vi "Dual XDCR AttnScan.vi"(0 "Length of\none plane (mm)":refnum<vi>, 1 "Distance between\nscan lines (um)":refnum<vi>, 3 "Case Name":refnum<vi>, 4 "DBSP2":refnum<vi>, 5 "DBSP1":refnum<vi>, 8 "Length of\nall planes (mm)":refnum<vi>, 9 "Scan Size":refnum<vi>, 10 "Length of Z Scan (mm)":dbl=5.0 format="%#_13g", 11 "Distance between\nZ planes (um)":i32=100, 12 "scan pair":T1=enum."y-(z) scan", 13 "Transducer":refnum<vi>, 14 "Attenuation Scan":bool, 15 "DBSP1":sgl, 17 "DBSP2":sgl, 19 "Dual XDCR Settings in":T2 {"XDCR Settings"."UT340 Controls"."Low Pass Filter (MHz)" min=-6 max=60 step=1; "XDCR Settings"."UT340 Controls"."High Pass Filter (MHz)" min=1 max=20 step=1; "XDCR Settings"."UT340 Controls"."Rep Rate (Hz)" min=20 step=1; "XDCR Settings"."UT340 Controls"."Pulse Width (ns)" min=100.0 max=250.0 step=2.0; "XDCR Settings"."UT340 Controls"."Voltage" min=100 max=250 step=2; "XDCR Settings"."UT340 Controls"."PC Gain (dB)" min=2 max=72; "XDCR Settings"."UT340 Controls"."PE Gain (dB)" min=-6 max=60 step=1; "XDCR Settings"."JSR Complete"."JSR Trigger Settings"."PRF (Hz)" items=["100 Hz"=0.1, "200 Hz"=0.2, "400 Hz"=0.4, "600 Hz"=0.6, "800 Hz"=0.8, "1000 Hz"=1.0, "1250 Hz"=1.25, "1500 Hz"=1.5, "1750 Hz"=1.75, "2000 Hz"=2.0, "2500 Hz"=2.5, "3000 Hz"=3.0, "3500 Hz"=3.5, "4000 Hz"=4.0, "4500 Hz"=4.5, "5000 Hz"=5.0]; "XDCR Settings"."JSR Complete"."JSR Trigger Settings"."Trigger Source" items=["Internal", "External"]; "XDCR Settings"."JSR Complete"."JSR Trigger Settings"."External Trigger Limit" items=["No Limit", "5 kHz"]; "XDCR Settings"."JSR Complete"."JSR Receive Settings"."Gain (dB)" min=-13 max=66 step=1; "XDCR Settings"."JSR Complete"."JSR Receive Settings"."Low Pass Filter" items=["5 MHz"=5, "10 MHz"=10, "15 MHz"=15, "22.5 MHz"=22, "35 MHz"=35, "50 MHz"=50]; "XDCR Settings"."JSR Complete"."JSR Receive Settings"."High Pass Filter" items=["DC"=0, "1 MHz"=1000, "2.5 MHz"=2500, "5 MHz"=5000, "7.5 MHz"=7500, "12.5 MHz"=12500]; "XDCR Settings"."JSR Complete"."JSR Receive Settings"."Receiver Mode" items=["Echo", "Through"]; "XDCR Settings"."JSR Complete"."JSR Pulse Settings"."Pulser Voltage (V)" items=["100"=100, "125"=125, "150"=150, "175"=175, "200"=200, "225"=225, "250"=250, "275"=275, "300"=300, "325"=325, "350"=350, "375"=375, "400"=400, "425"=425, "450"=450, "475"=475]; "XDCR Settings"."JSR Complete"."JSR Pulse Settings"."Pulser Impedance" items=["High z", "Low z"]; "XDCR Settings"."JSR Complete"."JSR Pulse Settings"."Pulse Energy Level" items=["0 (Minimum)", "1", "2", "3 (Maximum)"]; "XDCR Settings"."JSR Complete"."JSR Pulse Settings"."Damping" items=["331 Ohms"=331, "198 Ohms"=198, "142 Ohms"=142, "110 Ohms"=110, "92 Ohms"=92, "77 Ohms"=77, "67 Ohms"=67, "59 Ohms"=59, "52 Ohms"=52, "47 Ohms"=47, "43 Ohms"=43, "39 Ohms"=39, "37 Ohms"=37, "34 Ohms"=34, "32 Ohms"=32, "30 Ohms"=30]; "XDCR Settings"."Panametrics Settings"."FINE ATTENUATION" items=["00.0", "00.5", "01.0", "01.5", "02.0", "02.5", "03.0", "03.5", "04.0", "04.5", "05.0", "05.5", "06.0", "06.5", "07.0", "07.5", "08.0", "08.5", "09.0", "09.5", "10.0", "10.5", "11.0", "11.5", "12.0", "12.5", "13.0", "13.5", "14.0", "14.5", "15.0", "15.5"]; "XDCR Settings"."Panametrics Settings"."COARSE ATTENUATION" items=["00.0", "10.0", "20.0", "30.0", "40.0", "50.0"]; "XDCR Settings"."Panametrics Settings"."GAIN (db)" items=["26.0", "40.0", "54.0"]; "XDCR Settings"."Panametrics Settings"."PRF (KHz)" items=["XREMT", "EXBNC", "0.200", "0.500", "1.000", "2.000", "5.000", "10.00", "20.00"]; "XDCR Settings"."Panametrics Settings"."MODE" items=["P/ E", "THRU", "RPP", "EXT_PLSR"]; "XDCR Settings"."Panametrics Settings"."LP FILT (MHz)" items=["20", "50", "100", "200"]; "XDCR Settings"."Panametrics Settings"."HP FILT (KHz)" items=["1", "1000", "3000", "10000"]; "XDCR Settings"."Panametrics Settings"."DAMPING (Ohm)" items=["7", "10", "16", "20", "26", "30", "40", "50"]; "XDCR Settings"."Panametrics Settings"."ENERGY (uJ)" items=["1", "2", "4", "8", "16", "32"]; "XDCR Settings"."Daxsonics Settings"."Freq (MHz)" items=["4"=4, "5"=5, "6"=6, "8"=8, "10"=10, "12"=12, "14"=14, "15"=15, "16"=16, "17"=17, "18"=18, "20"=20, "25"=25, "30"=30, "35"=35, "40"=40, "45"=45, "50"=50]; "XDCR Settings"."Daxsonics Settings"."Voltage (V)" items=["0"=0, "5"=5, "10"=10, "15"=15, "20"=20, "25"=25, "30"=30, "35"=35, "40"=40, "45"=45, "50"=50, "55"=55, "60"=60, "65"=65, "70"=70, "75"=75, "80"=80, "85"=85, "90"=90, "95"=95, "100"=100, "110"=110, "120"=120, "130"=130, "140"=140, "150"=150, "160"=160, "170"=170, "180"=180, "190"=190]; "XDCR Settings"."Daxsonics Settings"."Gain (dB)" items=["22"=22, "25"=25, "28"=28, "31"=31, "34"=34, "37"=37, "40"=40, "43"=43, "46"=46, "49"=49, "52"=52, "55"=55, "58"=58, "61"=61, "64"=64, "67"=67]; "XDCR Settings"."Digitizer Settings"."Additional dig delay (ms)" format="%.2f"; "XDCR Settings"."Digitizer Settings"."Time scale per Div" items=["100 ns"=0.1, "200 ns"=0.2, "500 ns"=0.5, "1 micros"=1.0, "2 micros"=2.0, "5 micros"=5.0, "10 micros"=10.0, "20 micros"=20.0, "50 micros"=50.0, "100 micros"=100.0, "200 micros"=200.0, "500 micros"=500.0, "1 ms"=1000.0, "2 ms"=2000.0, "5 ms"=5000.0, "10 ms"=10000.0, "20 ms"=20000.0, "50 ms"=50000.0, "100 ms"=100000.0, "200 ms"=200000.0]; "XDCR Settings"."Digitizer Settings"."RF data Sampling"."rf points per line" min=1; "XDCR Settings"."Digitizer Settings"."RF data Sampling"."Ref Delay (ms)" format="%.2f"}) -> (16 "scan pair out":T1, 20 "lines per plane":dbl, 21 "Distance between\nscan lines (um)":sgl, 23 "number of planes":dbl, 24 "Distance between\nscan planes (um)":sgl, 25 "Dual XDCR Settings out":T2 {"XDCR Settings"."UT340 Controls"."Low Pass Filter (MHz)" min=-6 max=60 step=1; "XDCR Settings"."UT340 Controls"."High Pass Filter (MHz)" min=1 max=20 step=1; "XDCR Settings"."UT340 Controls"."Rep Rate (Hz)" min=20 step=1; "XDCR Settings"."UT340 Controls"."Pulse Width (ns)" min=100.0 max=250.0 step=2.0; "XDCR Settings"."UT340 Controls"."Voltage" min=100 max=250 step=2; "XDCR Settings"."UT340 Controls"."PC Gain (dB)" min=2 max=72; "XDCR Settings"."UT340 Controls"."PE Gain (dB)" min=-6 max=60 step=1; "XDCR Settings"."JSR Complete"."JSR Trigger Settings"."PRF (Hz)" items=["100 Hz"=0.1, "200 Hz"=0.2, "400 Hz"=0.4, "600 Hz"=0.6, "800 Hz"=0.8, "1000 Hz"=1.0, "1250 Hz"=1.25, "1500 Hz"=1.5, "1750 Hz"=1.75, "2000 Hz"=2.0, "2500 Hz"=2.5, "3000 Hz"=3.0, "3500 Hz"=3.5, "4000 Hz"=4.0, "4500 Hz"=4.5, "5000 Hz"=5.0]; "XDCR Settings"."JSR Complete"."JSR Trigger Settings"."Trigger Source" items=["Internal", "External"]; "XDCR Settings"."JSR Complete"."JSR Trigger Settings"."External Trigger Limit" items=["No Limit", "5 kHz"]; "XDCR Settings"."JSR Complete"."JSR Receive Settings"."Gain (dB)" min=-13 max=66 step=1; "XDCR Settings"."JSR Complete"."JSR Receive Settings"."Low Pass Filter" items=["5 MHz"=5, "10 MHz"=10, "15 MHz"=15, "22.5 MHz"=22, "35 MHz"=35, "50 MHz"=50]; "XDCR Settings"."JSR Complete"."JSR Receive Settings"."High Pass Filter" items=["DC"=0, "1 MHz"=1000, "2.5 MHz"=2500, "5 MHz"=5000, "7.5 MHz"=7500, "12.5 MHz"=12500]; "XDCR Settings"."JSR Complete"."JSR Receive Settings"."Receiver Mode" items=["Echo", "Through"]; "XDCR Settings"."JSR Complete"."JSR Pulse Settings"."Pulser Voltage (V)" items=["100"=100, "125"=125, "150"=150, "175"=175, "200"=200, "225"=225, "250"=250, "275"=275, "300"=300, "325"=325, "350"=350, "375"=375, "400"=400, "425"=425, "450"=450, "475"=475]; "XDCR Settings"."JSR Complete"."JSR Pulse Settings"."Pulser Impedance" items=["High z", "Low z"]; "XDCR Settings"."JSR Complete"."JSR Pulse Settings"."Pulse Energy Level" items=["0 (Minimum)", "1", "2", "3 (Maximum)"]; "XDCR Settings"."JSR Complete"."JSR Pulse Settings"."Damping" items=["331 Ohms"=331, "198 Ohms"=198, "142 Ohms"=142, "110 Ohms"=110, "92 Ohms"=92, "77 Ohms"=77, "67 Ohms"=67, "59 Ohms"=59, "52 Ohms"=52, "47 Ohms"=47, "43 Ohms"=43, "39 Ohms"=39, "37 Ohms"=37, "34 Ohms"=34, "32 Ohms"=32, "30 Ohms"=30]; "XDCR Settings"."Panametrics Settings"."FINE ATTENUATION" items=["00.0", "00.5", "01.0", "01.5", "02.0", "02.5", "03.0", "03.5", "04.0", "04.5", "05.0", "05.5", "06.0", "06.5", "07.0", "07.5", "08.0", "08.5", "09.0", "09.5", "10.0", "10.5", "11.0", "11.5", "12.0", "12.5", "13.0", "13.5", "14.0", "14.5", "15.0", "15.5"]; "XDCR Settings"."Panametrics Settings"."COARSE ATTENUATION" items=["00.0", "10.0", "20.0", "30.0", "40.0", "50.0"]; "XDCR Settings"."Panametrics Settings"."GAIN (db)" items=["26.0", "40.0", "54.0"]; "XDCR Settings"."Panametrics Settings"."PRF (KHz)" items=["XREMT", "EXBNC", "0.200", "0.500", "1.000", "2.000", "5.000", "10.00", "20.00"]; "XDCR Settings"."Panametrics Settings"."MODE" items=["P/ E", "THRU", "RPP", "EXT_PLSR"]; "XDCR Settings"."Panametrics Settings"."LP FILT (MHz)" items=["20", "50", "100", "200"]; "XDCR Settings"."Panametrics Settings"."HP FILT (KHz)" items=["1", "1000", "3000", "10000"]; "XDCR Settings"."Panametrics Settings"."DAMPING (Ohm)" items=["7", "10", "16", "20", "26", "30", "40", "50"]; "XDCR Settings"."Panametrics Settings"."ENERGY (uJ)" items=["1", "2", "4", "8", "16", "32"]; "XDCR Settings"."Daxsonics Settings"."Freq (MHz)" items=["4"=4, "5"=5, "6"=6, "8"=8, "10"=10, "12"=12, "14"=14, "15"=15, "16"=16, "17"=17, "18"=18, "20"=20, "25"=25, "30"=30, "35"=35, "40"=40, "45"=45, "50"=50]; "XDCR Settings"."Daxsonics Settings"."Voltage (V)" items=["0"=0, "5"=5, "10"=10, "15"=15, "20"=20, "25"=25, "30"=30, "35"=35, "40"=40, "45"=45, "50"=50, "55"=55, "60"=60, "65"=65, "70"=70, "75"=75, "80"=80, "85"=85, "90"=90, "95"=95, "100"=100, "110"=110, "120"=120, "130"=130, "140"=140, "150"=150, "160"=160, "170"=170, "180"=180, "190"=190]; "XDCR Settings"."Daxsonics Settings"."Gain (dB)" items=["22"=22, "25"=25, "28"=28, "31"=31, "34"=34, "37"=37, "40"=40, "43"=43, "46"=46, "49"=49, "52"=52, "55"=55, "58"=58, "61"=61, "64"=64, "67"=67]; "XDCR Settings"."Digitizer Settings"."Additional dig delay (ms)" format="%.2f"; "XDCR Settings"."Digitizer Settings"."Time scale per Div" items=["100 ns"=0.1, "200 ns"=0.2, "500 ns"=0.5, "1 micros"=1.0, "2 micros"=2.0, "5 micros"=5.0, "10 micros"=10.0, "20 micros"=20.0, "50 micros"=50.0, "100 micros"=100.0, "200 micros"=200.0, "500 micros"=500.0, "1 ms"=1000.0, "2 ms"=2000.0, "5 ms"=5000.0, "10 ms"=10000.0, "20 ms"=20000.0, "50 ms"=50000.0, "100 ms"=100000.0, "200 ms"=200000.0]; "XDCR Settings"."Digitizer Settings"."RF data Sampling"."rf points per line" min=1; "XDCR Settings"."Digitizer Settings"."RF data Sampling"."Ref Delay (ms)" format="%.2f"})   [LabVIEW 2022 SP3]
uses:
  Dual XDCR Complete Settings.ctl
  XDCRSettings.ctl
  Pulsers/Daxsonics/-DaxSubroutines/Dax_Control_Cluster.ctl
  Pulsers/Panametrics/Pana5900.ctl
  Pulsers/JSR/Controls/JSR Complete.ctl
  Pulsers/JSR/Controls/JSR Pulse.ctl
  Pulsers/JSR/Controls/Damping.ctl
  Pulsers/JSR/Controls/Energy.ctl
  Pulsers/JSR/Controls/Z.ctl
  Pulsers/JSR/Controls/Volt.ctl
  Pulsers/JSR/Controls/JSR Recieve.ctl
  Pulsers/JSR/Controls/Mode.ctl
  Pulsers/JSR/Controls/HPF.ctl
  Pulsers/JSR/Controls/LPF.ctl
  Pulsers/JSR/Controls/Gain.ctl
  Pulsers/JSR/Controls/JSR Trigger.ctl
  Pulsers/JSR/Controls/Trig Limit.ctl
  Pulsers/JSR/Controls/Trig Source.ctl
  Pulsers/JSR/Controls/PRF.ctl
  Pulsers/UTEX/Controls/UTEX Controls.ctl
  Motion Controllers/-MotionRoutines/ScanAxis.ctl
  <vilib>/regexp/Match Regular Expression.xnode
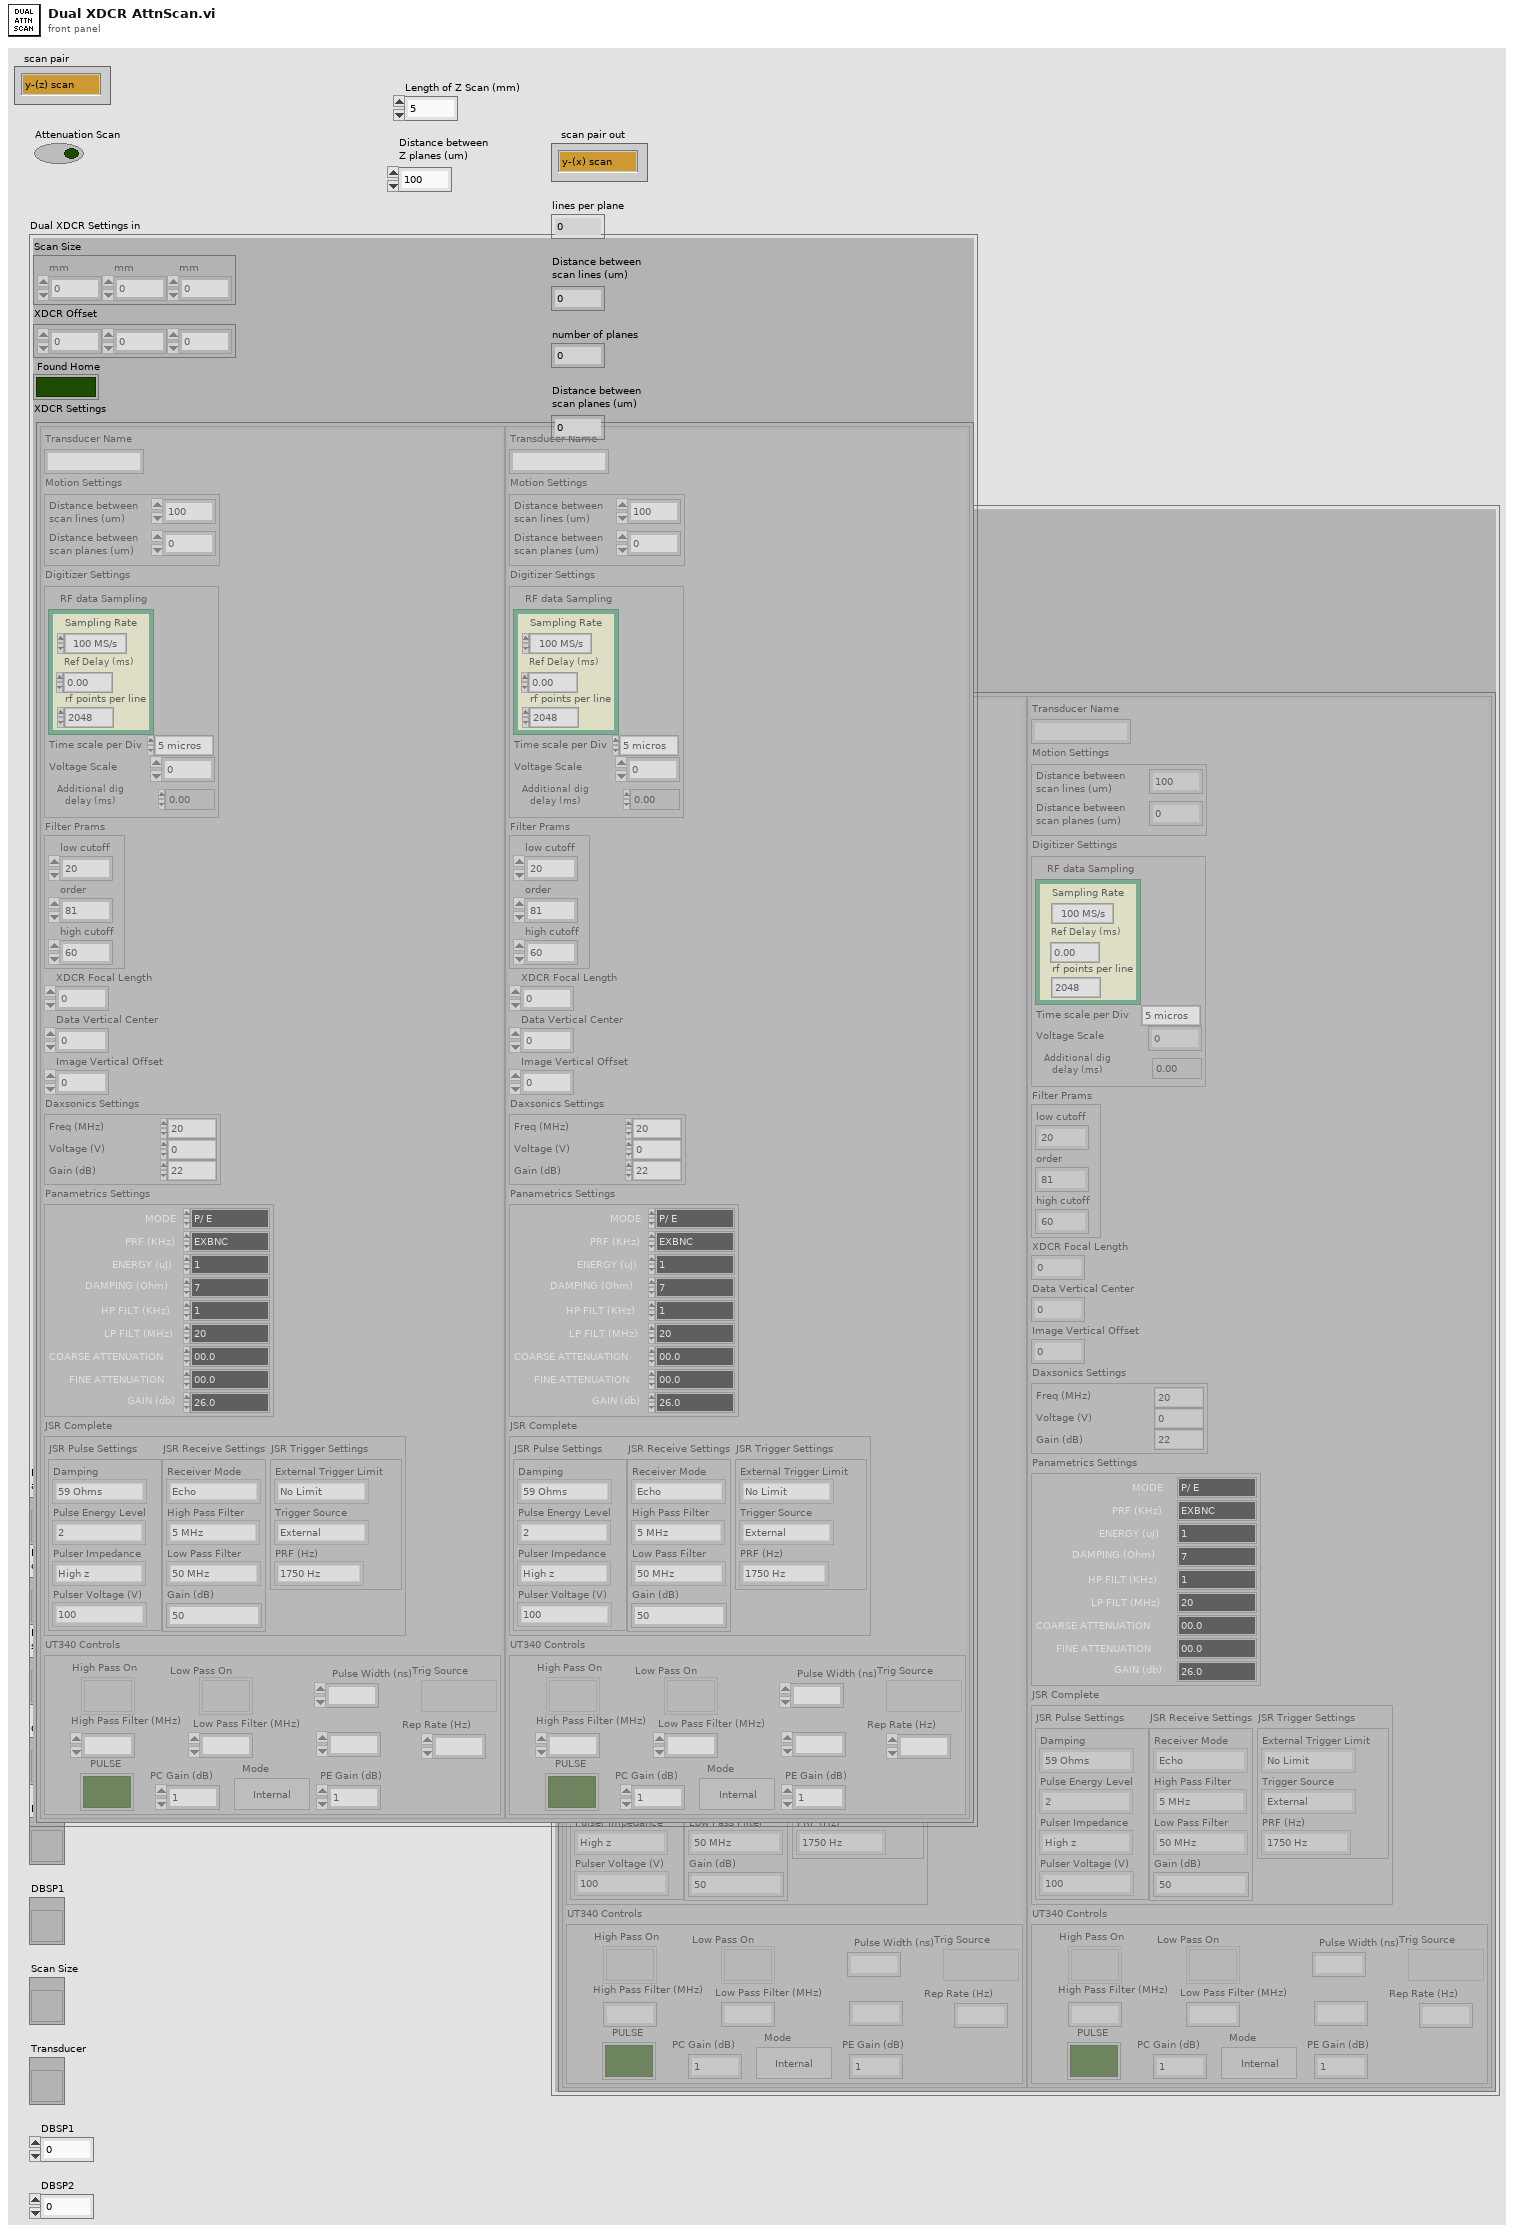
[diagram p1: front panel]
types:
  T1 = typedef "ScanAxis.ctl" = enum16{"y-(x) scan", "x-(y) scan", "z-(x) scan", "z-(y) scan", "y-(z) scan", "x-(z) scan", "w-(x) scan", "w-(y) scan", "w-(z) scan", "x-(w) scan", "y-(w) scan", "z-(w) scan"}
  T2 = typedef "Dual XDCR Complete Settings.ctl" = cluster{"Scan Size":dbl[], "XDCR Offset":dbl[], "Found Home":bool, "XDCR Settings":T3[]}
  T3 = typedef "XDCRSettings.ctl" = cluster{"Transducer Name":string, "Motion Settings":cluster{"Distance between\nscan lines (um)":sgl, "Distance between\nscan planes (um)":sgl}, "Digitizer Settings":cluster{"RF data Sampling":cluster{"Sampling Rate":dbl, "Ref Delay (ms)":dbl, "rf points per line":i32}, "Time scale per Div":dbl, "Voltage Scale":dbl, "Additional dig delay (ms)":dbl}, "Filter Prams":cluster{"low cutoff":i32, "order":i32, "high cutoff":i32}, "XDCR Focal Length":dbl, "Data Vertical Center":dbl, "Image Vertical Offset":dbl, "Daxsonics Settings":T4, "Panametrics Settings":T5, "JSR Complete":T6, "UT340 Controls":T21}
  T4 = typedef "Dax_Control_Cluster.ctl" = cluster{"Freq (MHz) ":u16, "Voltage (V)":u16, "Gain (dB)":u16}
  T5 = typedef "Pana5900.ctl" = cluster{"ENERGY (uJ)":u16, "DAMPING (Ohm)":u16, "HP FILT (KHz) ":u16, "LP FILT (MHz)":u16, "MODE":u16, "PRF (KHz)":u16, "GAIN (db)":u16, "COARSE ATTENUATION":u16, "FINE ATTENUATION":u16}
  T6 = typedef "JSR Complete.ctl" = cluster{"JSR Pulse Settings":T7, "JSR Receive Settings":T12, "JSR Trigger Settings":T17}
  T7 = typedef "JSR Pulse.ctl" = cluster{"Damping":T8, "Pulse Energy Level":T9, "Pulser Impedance":T10, "Pulser Voltage (V)":T11}
  T8 = typedef "Damping.ctl" = i16
  T9 = typedef "Energy.ctl" = u16
  T10 = typedef "Z.ctl" = u16
  T11 = typedef "Volt.ctl" = i16
  T12 = typedef "JSR Recieve.ctl" = cluster{"Receiver Mode":T13, "High Pass Filter":T14, "Low Pass Filter":T15, "Gain (dB)":T16}
  T13 = typedef "Mode.ctl" = i8
  T14 = typedef "HPF.ctl" = u16
  T15 = typedef "LPF.ctl" = u16
  T16 = typedef "Gain.ctl" = i8
  T17 = typedef "JSR Trigger.ctl" = cluster{"External Trigger Limit":T18, "Trigger Source":T19, "PRF (Hz)":T20}
  T18 = typedef "Trig Limit.ctl" = i8
  T19 = typedef "Trig Source.ctl" = i8
  T20 = typedef "PRF.ctl" = dbl
  T21 = typedef "UTEX Controls.ctl" = cluster{"High Pass On":bool, "High Pass Filter (MHz)":i16, "Low Pass On":bool, "Low Pass Filter (MHz)":i16, "PE Gain (dB)":i16, "Voltage":i16, "Pulse Width (ns)":dbl, "Mode":bool, "PC Gain (dB)":i16, "Trig Source":bool, "Rep Rate (Hz)":i16, "PULSE":bool}
  T22 = cluster{"Distance between\nscan lines (um)":sgl, "Distance between\nscan planes (um)":sgl}
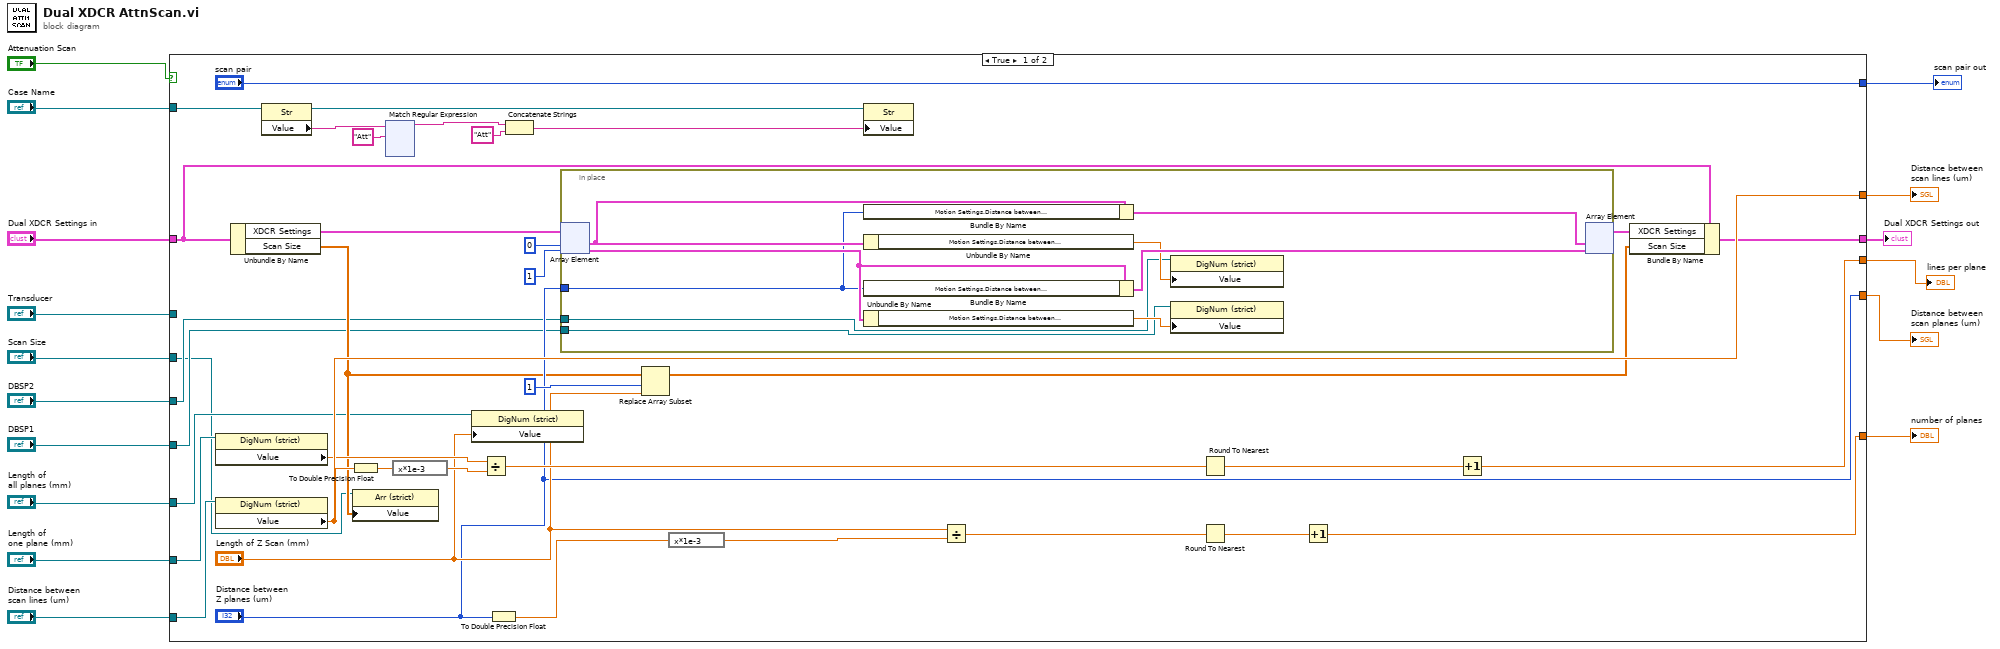
[diagram p0: block diagram]
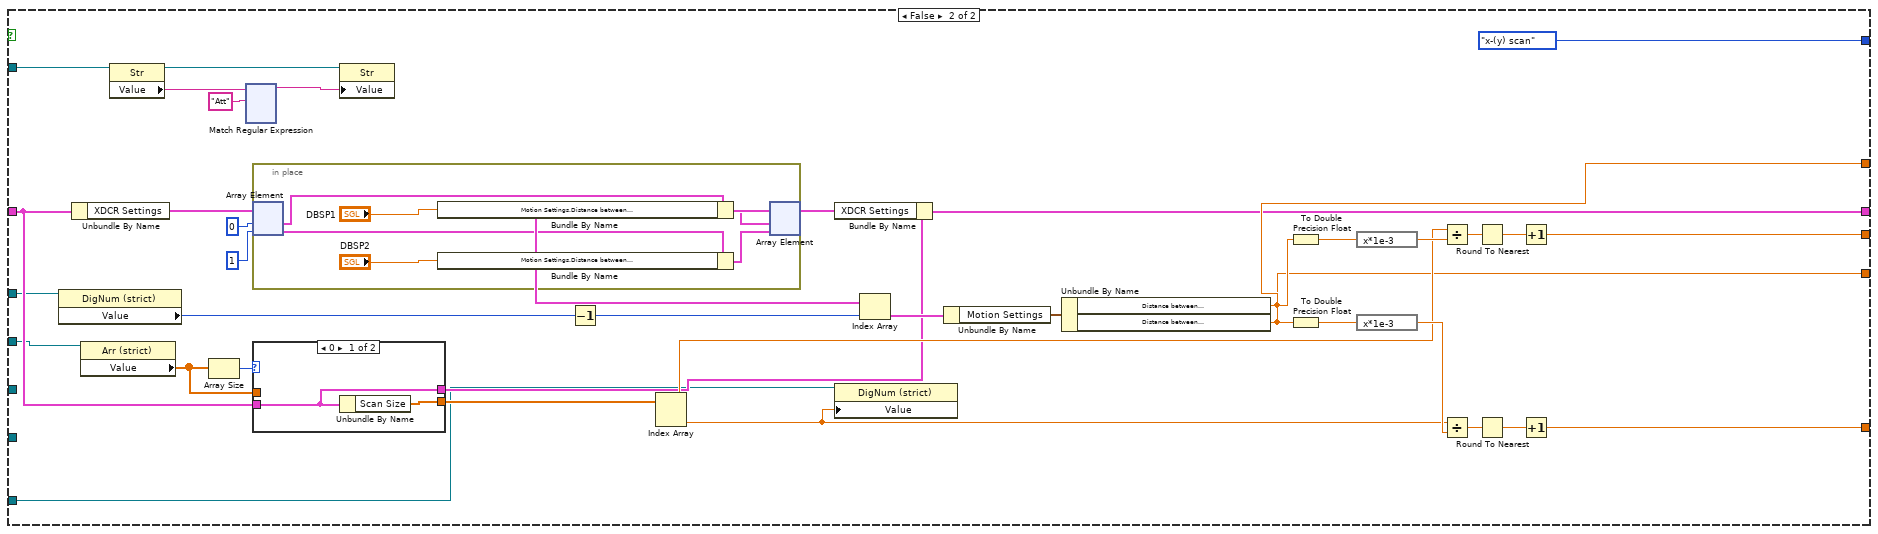
[diagram p2: hidden frame]
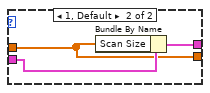
[diagram p3: hidden frame]
diagram:
  n1 = case shown="True" "Attenuation Scan" {
    tunnel: [w53 w216] -> w9
    tunnel: ["scan pair" ScanAxis."x-(y) scan" ("scan pair")] -> w10
    tunnel: [w51 w196] -> w11
    tunnel: ["Distance between\nZ planes (um)" w195] -> w12
    tunnel: [w50 w214] -> w13
    tunnel: "Dual XDCR Settings in" -> [w38 w194]
    tunnel: [w34 w186] -> w15
    tunnel: "Length of\none plane (mm)" -> [w27 _]
    tunnel: "Length of\nall planes (mm)" -> [w26 w180]
    tunnel: "Distance between\nscan lines (um)" -> [w25 _]
    tunnel: "DBSP2" -> [w24 _]
    tunnel: "DBSP1" -> [w23 _]
    tunnel: "Case Name" -> [w19 w184]
    tunnel: "Transducer" -> [_ w183]
    tunnel: "Scan Size" -> [w22 w182]
    frame True {
      n2 = property on="Property Node" class="DigNum (strict)"(reference=w27) -> ("Value"=w45:dbl)  [unwired: 1 in, 2 out]
      n3 = property on="Property Node" class="DigNum (strict)"(reference=w25) -> ("Value"=w51:sgl)  [unwired: 1 in, 2 out]
      n4 = Unbundle By Name(w38) -> ("XDCR Settings"=w33:T3[], "Scan Size"=w28:dbl[])
      n5 = property on="Property Node" class="Str"(reference=w19) -> (reference out=w18:refnum<vi>, "Value"=w21:string)  [unwired: 1 in, 1 out]
      n6 = To Double Precision Float(number=w51) -> (double precision float=w47:dbl)
      n7 = property on="Property Node" class="Arr (strict)"(reference=w22, "Value"=w28) -> ()  [unwired: 1 in, 2 out]
      n8 = xnode "Match Regular Expression"("input string"=w21, "regular expression"="Att" ("string")) -> ("before match"=w17:string)  [unwired: 4 in, 4 out]
      n9 = expression code="x*1e-3"(w47) -> (w48:dbl)
      n10 = property on="Property Node" class="DigNum (strict)"(reference=w26, "Value"="Length of Z Scan (mm)") -> ()  [unwired: 1 in, 2 out]
      n11 = Divide(x=w45, y=w48) -> (x/y=w49:dbl)
      n12 = To Double Precision Float(number="Distance between\nZ planes (um)") -> (double precision float=w42:dbl)
      n13 = Concatenate Strings(w17, "Att" ("string")) -> (w40:string)
      n14 = in-place {
        in-place-border: "Distance between\nZ planes (um)" -> [w175]
        in-place-border: w24 -> [w172]
        in-place-border: w23 -> [w171]
        n15 = in-place-array #1(w33, 0, 1) -> (w178:T3, w176:T3)
        n16 = Bundle By Name(cluster=w178, "Motion Settings.Distance between\nscan planes (um)"=w175) -> (w179:T3)
        n17 = Unbundle By Name(w178) -> ("Motion Settings.Distance between\nscan planes (um)"=w174:sgl)
        n18 = Bundle By Name(cluster=w176, "Motion Settings.Distance between\nscan planes (um)"=w175) -> (w177:T3)
        n19 = Unbundle By Name(w176) -> ("Motion Settings.Distance between\nscan planes (um)"=w173:sgl)
        n20 = property on="Property Node" class="DigNum (strict)"(reference=w172, "Value"=w174) -> ()  [unwired: 1 in, 2 out]
        n21 = property on="Property Node" class="DigNum (strict)"(reference=w171, "Value"=w173) -> ()  [unwired: 1 in, 2 out]
        n22 = in-place-array #1(w179, w177) -> (w32:T3[])  [unwired: 2 out]
      }
      n23 = Replace Array Subset(array=w28, new element="Length of Z Scan (mm)", index=1) -> (w37:dbl[])
      n24 = expression code="x*1e-3"(w42) -> (w43:dbl)
      n25 = property on="Property Node" class="Str"(reference=w18, "Value"=w40) -> ()  [unwired: 1 in, 2 out]
      n26 = Divide(x="Length of Z Scan (mm)", y=w43) -> (x/y=w44:dbl)
      n27 = Round To Nearest(number=w49) -> (nearest integer value=w46:dbl)
      n28 = Round To Nearest(number=w44) -> (nearest integer value=w41:dbl)
      n29 = Increment(x=w41) -> (x+1=w53:dbl)
      n30 = Increment(x=w46) -> (x+1=w50:dbl)
      n31 = Bundle By Name(cluster=w38, "XDCR Settings"=w32, "Scan Size"=w37) -> (w34:T2)
    }
    frame False {
      n32 = property on="Property Node" class="DigNum (strict)"(reference=w183) -> ("Value"=w201:u32)  [unwired: 1 in, 2 out]
      n33 = Unbundle By Name(w194) -> ("XDCR Settings"=w187:T3[])
      n34 = property on="Property Node" class="Arr (strict)"(reference=w182) -> ("Value"=w191:dbl[])  [unwired: 1 in, 2 out]
      n35 = property on="Property Node" class="Str"(reference=w184) -> (reference out=w181:refnum<vi>, "Value"=w205:string)  [unwired: 1 in, 1 out]
      n36 = Array Size(array=w191) -> (size(s)=w192:i32)
      n37 = xnode "Match Regular Expression"("input string"=w205, "regular expression"="Att" ("string")) -> ("before match"=w203:string)  [unwired: 4 in, 4 out]
      n38 = in-place {
        n39 = in-place-array #2(w187, 0, 1) -> (w221:T3, w219:T3)
        n40 = Bundle By Name(cluster=w221, "Motion Settings.Distance between\nscan planes (um)"="DBSP1") -> (w222:T3)
        n41 = Bundle By Name(cluster=w219, "Motion Settings.Distance between\nscan planes (um)"="DBSP2") -> (w220:T3)
        n42 = in-place-array #2(w222, w220) -> (w185:T3[])  [unwired: 2 out]
      }
      n43 = case shown="0" w192 {
        tunnel: w194 -> [w223 w227]
        tunnel: [w223 w226] -> w193
        tunnel: w191 -> [_ w225]
        tunnel: [w224 w225] -> w190
        frame 0 {
          n44 = Unbundle By Name(w223) -> ("Scan Size"=w224:dbl[])
        }
        frame 1, Default {
          n45 = Bundle By Name(cluster=w227, "Scan Size"=w225) -> (w226:T2)
        }
      }
      n46 = property on="Property Node" class="Str"(reference=w181, "Value"=w203) -> ()  [unwired: 1 in, 2 out]
      n47 = Decrement(x=w201) -> (x-1=w202:u32)
      n48 = Index Array(array=w190) -> (element #1=w200:dbl, element #2=w199:dbl)  [unwired: 2 in]
      n49 = Bundle By Name(cluster=w193, "XDCR Settings"=w185) -> (w186:T2)
      n50 = property on="Property Node" class="DigNum (strict)"(reference=w180, "Value"=w199) -> ()  [unwired: 1 in, 2 out]
      n51 = Index Array(array=w185, index=w202) -> (element=w198:T3)
      n52 = Unbundle By Name(w198) -> ("Motion Settings"=w197:T22)
      n53 = Unbundle By Name(w197) -> ("Distance between\nscan lines (um)"=w196:sgl, "Distance between\nscan planes (um)"=w195:sgl)
      n54 = To Double Precision Float(number=w196) -> (double precision float=w211:dbl)
      n55 = To Double Precision Float(number=w195) -> (double precision float=w207:dbl)
      n56 = expression code="x*1e-3"(w211) -> (w212:dbl)
      n57 = expression code="x*1e-3"(w207) -> (w208:dbl)
      n58 = Divide(x=w200, y=w212) -> (x/y=w213:dbl)
      n59 = Divide(x=w199, y=w208) -> (x/y=w209:dbl)
      n60 = Round To Nearest(number=w213) -> (nearest integer value=w210:dbl)
      n61 = Round To Nearest(number=w209) -> (nearest integer value=w206:dbl)
      n62 = Increment(x=w210) -> (x+1=w214:dbl)
      n63 = Increment(x=w206) -> (x+1=w216:dbl)
    }
  }
  "Dual XDCR Settings out" <- w15
  "lines per plane" <- w13
  "Distance between\nscan planes (um)" <- w12
  "Distance between\nscan lines (um)" <- w11
  "scan pair out" <- w10
  "number of planes" <- w9
